vi "DB - Split DB.Schema.Table.vi"(10 "DB.Schema.Table String":string[](array[string])) -> (2 "DB Schema Table DS":T1[](array[typedef]))   [LabVIEW 2020]
uses:
  Control/DB Schema Table DS.ctl
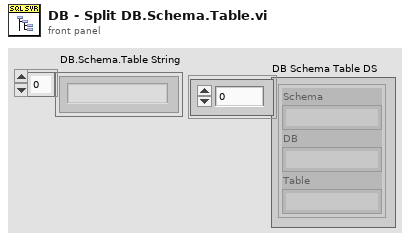
[diagram p1: front panel]
types:
  T1 = typedef "DB Schema Table DS.ctl" = cluster{"Schema":string, "DB":string, "Table":string}
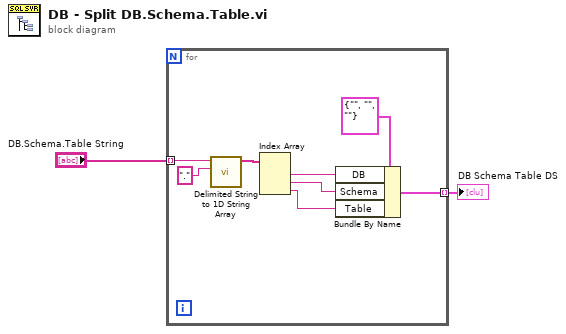
[diagram p0: block diagram]
diagram:
  n1 = for {
    tunnel: "DB.Schema.Table String" -> [w9] mode=indexing
    tunnel: [w3] -> w1 mode=indexing
    n2 = call <vilib>:"Delimited String to 1D String Array.vi"("delimiter"=".", "delimited string"=w9) -> ("string array"=w7:string[])  [unwired: 9 in]
    n3 = Index Array(array=w7) -> (element #1=w6:string, element #2=w5:string, element #3=w4:string)  [unwired: 3 in]
    n4 = Bundle By Name(cluster=T1 {"Schema"="", "DB"="", "Table"=""} ("DB.Schema.Table"), "DB"=w6, "Schema"=w5, "Table"=w4) -> (w3:T1)
  }
  "DB Schema Table DS" <- w1
